vi "RichToFlatni_measurementlink_measurement_v1_MeasurementSignature.vi"(5 "OutputClusterType":T1, 11 "InputCluster":T7) -> (3 "OutputCluster":T1)   [LabVIEW 2020, in "Measurement Plugin Measurement Server Internal.lvlib"]
uses:
  Measurement Plugin Measurement Server Internal.lvlib
  ni_measurementlink_measurement_v1_MeasurementSignature.ctl
  ni_measurementlink_measurement_v1_ConfigurationParameter.ctl
  google_protobuf_Field_Kind.ctl
  ni_measurementlink_measurement_v1_ConfigurationParameter_AnnotationsEntry.ctl
  google_protobuf_Any.ctl
  ni_measurementlink_measurement_v1_Output.ctl
  ni_measurementlink_measurement_v1_MeasurementSignature_Flat.ctl
  ni_measurementlink_measurement_v1_ConfigurationParameter_Flat.ctl
  ni_measurementlink_measurement_v1_ConfigurationParameter_AnnotationsEntry_Flat.ctl
  google_protobuf_Any_Flat.ctl
  ni_measurementlink_measurement_v1_Output_Flat.ctl
  RichToFlatni_measurementlink_measurement_v1_ConfigurationParameter_AnnotationsEntry.vi
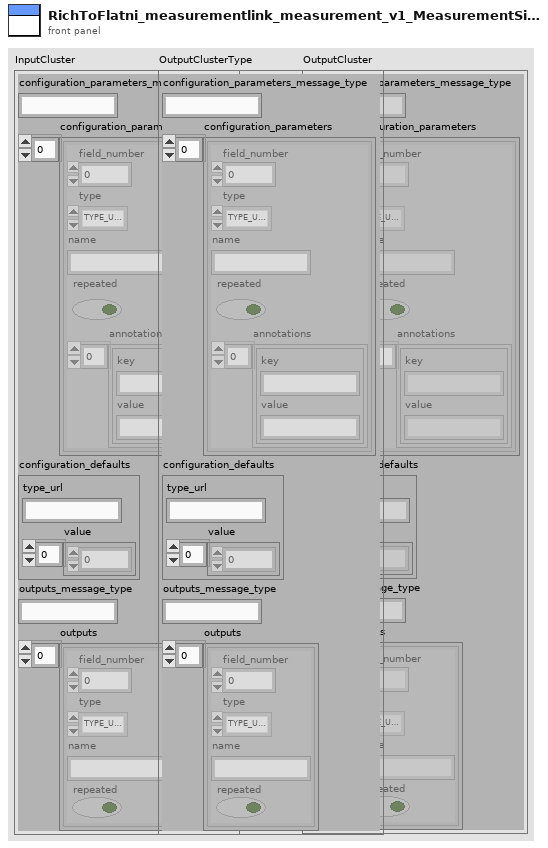
[diagram p1: front panel]
types:
  T1 = typedef "Measurement Plugin Measurement Server Internal.lvlib/ni_measurementlink_measurement_v1_MeasurementSignature_Flat.ctl" = cluster{"configuration_parameters_message_type":string, "configuration_parameters":T2[], "configuration_defaults":T5, "outputs_message_type":string, "outputs":T6[]}
  T2 = typedef "Measurement Plugin Measurement Server Internal.lvlib/ni_measurementlink_measurement_v1_ConfigurationParameter_Flat.ctl" = cluster{"field_number":i32, "type":T3, "name":string, "repeated":bool, "annotations":T4[]}
  T3 = typedef "Measurement Plugin Measurement Server Internal.lvlib/google_protobuf_Field_Kind.ctl" = enum32{"TYPE_UNKNOWN", "TYPE_DOUBLE", "TYPE_FLOAT", "TYPE_INT64", "TYPE_UINT64", "TYPE_INT32", "TYPE_FIXED64", "TYPE_FIXED32", "TYPE_BOOL", "TYPE_STRING", "TYPE_GROUP", "TYPE_MESSAGE", "TYPE_BYTES", "TYPE_UINT32", "TYPE_ENUM", "TYPE_SFIXED32", "TYPE_SFIXED64", "TYPE_SINT32", "TYPE_SINT64"}
  T4 = typedef "Measurement Plugin Measurement Server Internal.lvlib/ni_measurementlink_measurement_v1_ConfigurationParameter_AnnotationsEntry_Flat.ctl" = cluster{"key":string, "value":string}
  T5 = typedef "Measurement Plugin Measurement Server Internal.lvlib/google_protobuf_Any_Flat.ctl" = cluster{"type_url":string, "value":u8[]}
  T6 = typedef "Measurement Plugin Measurement Server Internal.lvlib/ni_measurementlink_measurement_v1_Output_Flat.ctl" = cluster{"field_number":i32, "type":T3, "name":string, "repeated":bool}
  T7 = typedef "Measurement Plugin Measurement Server Internal.lvlib/ni_measurementlink_measurement_v1_MeasurementSignature.ctl" = cluster{"configuration_parameters_message_type":string, "configuration_parameters":T8[], "configuration_defaults":T10, "outputs_message_type":string, "outputs":T11[]}
  T8 = typedef "Measurement Plugin Measurement Server Internal.lvlib/ni_measurementlink_measurement_v1_ConfigurationParameter.ctl" = cluster{"field_number":i32, "type":T3, "name":string, "repeated":bool, "annotations":T9[]}
  T9 = typedef "Measurement Plugin Measurement Server Internal.lvlib/ni_measurementlink_measurement_v1_ConfigurationParameter_AnnotationsEntry.ctl" = cluster{"key":string, "value":string}
  T10 = typedef "Measurement Plugin Measurement Server Internal.lvlib/google_protobuf_Any.ctl" = cluster{"type_url":string, "value":u8[]}
  T11 = typedef "Measurement Plugin Measurement Server Internal.lvlib/ni_measurementlink_measurement_v1_Output.ctl" = cluster{"field_number":i32, "type":T3, "name":string, "repeated":bool}
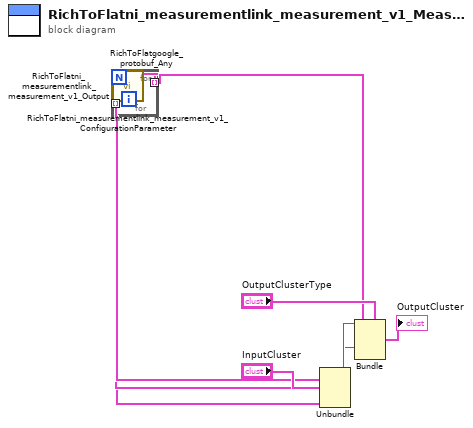
[diagram p0: block diagram]
diagram:
  n1 = Unbundle "Unbundle"("InputCluster") -> ("configuration_parameters_message_type"=w8:string, "configuration_parameters"=w7:T8[], "configuration_defaults"=w5:T10, "outputs_message_type"=w3:string, "outputs"=w2:T11[])
  n2 = for {
    tunnel: w2 -> [w13] mode=indexing
    tunnel: [w12] -> w1 mode=indexing
    n3 = call "RichToFlatni_measurementlink_measurement_v1_Output.vi"("InputCluster"=w13) -> ("OutputCluster"=w12:T6)  [unwired: 10 in]
  }
  n4 = call "RichToFlatgoogle_protobuf_Any.vi"("InputCluster"=w5) -> ("OutputCluster"=w4:T5)  [unwired: 10 in]
  n5 = for {
    tunnel: w7 -> [w15] mode=indexing
    tunnel: [w14] -> w6 mode=indexing
    n6 = call "RichToFlatni_measurementlink_measurement_v1_ConfigurationParameter.vi"("InputCluster"=w15) -> ("OutputCluster"=w14:T2)  [unwired: 10 in]
  }
  n7 = Bundle "Bundle"(cluster="OutputClusterType", "configuration_parameters_message_type"=w8, "configuration_parameters"=w6, "configuration_defaults"=w4, "outputs_message_type"=w3, "outputs"=w1) -> (→"OutputCluster":T1)
